vi "Xml_Load_Expert.vi"(7 "Version String":string, 8 "error in (no error)":errorcluster, 10 "XML Path":path=path "D:/TEST.xml", 11 "Refnum Clust":refnum<vi>) -> (0 "error out":errorcluster)   [LabVIEW 2024]
uses:
  controls/SOFTWARE_Inputs.ctl
  controls/HARDWARE_Inputs.ctl
  controls/AO_6711_Inputs.ctl
  controls/AO_6738_Inputs.ctl
  controls/AWG_5421_Inputs.ctl
  <instrlib>/niFgen/niFgen.llb/niFgen_ctl Trigger Source Values (Ring).ctl
  controls/DIGIT_5122_Inputs.ctl
  <instrlib>/niScope/Controls/niScope trigger source.ctl
  controls/HSDIO_6541_Inputs.ctl
  <instrlib>/niHSDIO/niHSDIO.llb/niHSDIO_ctl Trigger Source Values (Ring).ctl
  controls/EXPERT_Inputs.ctl
  controls/XML_Inputs.ctl
panel:
  in  "EXPERT Inputs":T1={"XML Inputs"={"Version Tag Name"="XML_Version", "Version String"="1.0"}, "SOFTWARE Inputs"={"Application Directory"=path "D:/S.O.F.T.S/LABVIEW/PIL", "Software Version"="1.0.0", "Data Path"=path "D:/PIRENEA/DATA", "XML Path"=path "D:/PIRENEA/DATA", "XML File Filter"="*.xml", "XML Saved Path"=path "D:/PIRENEA/DATA/SAVED", "Excit Scripts Path"=path "D:/PIRENEA/EXCIT_SCRIPTS", "Excit Scripts File Filter"="*.txt", "Excit Waveforms Path"=path "D:/PIRENEA/EXCIT_WFMS", "Excit Waveforms File Filter"="*.bin", "Timing Scripts Path"=path "D:/PIRENEA/TIMING_SCRIPTS", "Timing Scripts File Filter"="*.txt", "Timing Waveforms Path"=path "D:/PIRENEA/TIMING_WFMS", "Timing Waveforms File Filter"="*.bin", "Trapping Waveforms Path"=path "D:/PIRENEA/TRAPPING_WFMS", "Trapping Waveforms File Filter"="*.bin"}, "HSDIO 6541 Inputs"={"Resource Name"="HSDIO_6541", "Clock Rate"=1000000.0, "Trigger Source"="PFI0"}, "AWG 5421 Inputs"={"Resource Name"="AWG_5421", "Sample Rate"=10000000.0, "Trigger Type"=2, "Trigger Source"="PFI0", "Waveform Gain"=0.31, "Digital Filter ON"=TRUE}, "DIGIT 5122 Inputs"={"Sample Rate"=10000.0, "Resource Name"="DIGIT_5122", "Channel Name"="0", "Trigger Source"="VAL_EXTERNAL", "Vertical Range"=10.0, "Trigger Level"=3.0}, "AO 6711 Inputs"={"Physical Channels"="AO_6711/ao0:3", "Min Voltage"=-10.0, "Max Voltage"=10.0, "Trigger Source"="/AO_6711/PFI3", "Counter"="AO_6711/ctr0"}, "AO 6738 Inputs"={"Physical Channels"="AO_6738/ao0:3", "Min Voltage"=-10.0, "Max Voltage"=10.0, "Trigger Source"="/AO_6738/PFI2", "Counter"="AO_6738/ctr0"}} {"AO 6738 Inputs"."Max Voltage" min=-10.0 max=10.0; "AO 6738 Inputs"."Min Voltage" min=-10.0 max=10.0; "AWG 5421 Inputs"."Sample Rate" format="%.2p"; "AWG 5421 Inputs"."Trigger Type" items=["None", "Software Edge", "Digital Edge", "Digital Level"]; "AO 6711 Inputs"."Max Voltage" min=-10.0 max=10.0; "AO 6711 Inputs"."Min Voltage" min=-10.0 max=10.0; "HSDIO 6541 Inputs"."Clock Rate" format="%.2p"; "DIGIT 5122 Inputs"."Trigger Level" format="%.2f"; "DIGIT 5122 Inputs"."Vertical Range" format="%.2f"; "DIGIT 5122 Inputs"."Sample Rate" step=65535.0 format="%#_3p"}
  in  "HARDWARE Inputs":T12={"AO 6711 Inputs"={"Physical Channels"="AO_6711/ao0:3", "Min Voltage"=-10.0, "Max Voltage"=10.0, "Trigger Source"="/AO_6711/PFI3", "Counter"="AO_6711/ctr0"}, "AO 6738 Inputs"={"Physical Channels"="AO_6738/ao0:3", "Min Voltage"=-10.0, "Max Voltage"=10.0, "Trigger Source"="/AO_6738/PFI2", "Counter"="AO_6738/ctr0"}, "AWG 5421 Inputs"={"Resource Name"="AWG_5421", "Sample Rate"=10000000.0, "Trigger Type"=2, "Trigger Source"="PFI0", "Waveform Gain"=0.31, "Digital Filter ON"=TRUE}, "DIGIT 5122 Inputs"={"Sample Rate"=10000.0, "Resource Name"="DIGIT_5122", "Channel Name"="0", "Trigger Source"="VAL_EXTERNAL", "Vertical Range"=10.0, "Trigger Level"=3.0}, "HSDIO 6541 Inputs"={"Resource Name"="HSDIO_6541", "Clock Rate"=1000000.0, "Trigger Source"="PFI0"}} {"AO 6738 Inputs"."Max Voltage" min=-10.0 max=10.0; "AO 6738 Inputs"."Min Voltage" min=-10.0 max=10.0; "HSDIO 6541 Inputs"."Clock Rate" format="%.2p"; "DIGIT 5122 Inputs"."Trigger Level" format="%.2f"; "DIGIT 5122 Inputs"."Vertical Range" format="%.2f"; "DIGIT 5122 Inputs"."Sample Rate" step=65535.0 format="%#_3p"; "AWG 5421 Inputs"."Sample Rate" format="%.2p"; "AWG 5421 Inputs"."Trigger Type" items=["None", "Software Edge", "Digital Edge", "Digital Level"]; "AO 6711 Inputs"."Max Voltage" min=-10.0 max=10.0; "AO 6711 Inputs"."Min Voltage" min=-10.0 max=10.0}
  in  "SOFTWARE Inputs":T3={"Application Directory"=path "D:/S.O.F.T.S/LABVIEW/PIL", "Software Version"="1.0.0", "Data Path"=path "D:/PIRENEA/DATA", "XML Path"=path "D:/PIRENEA/DATA", "XML File Filter"="*.xml", "XML Saved Path"=path "D:/PIRENEA/DATA/SAVED", "Excit Scripts Path"=path "D:/PIRENEA/EXCIT_SCRIPTS", "Excit Scripts File Filter"="*.txt", "Excit Waveforms Path"=path "D:/PIRENEA/EXCIT_WFMS", "Excit Waveforms File Filter"="*.bin", "Timing Scripts Path"=path "D:/PIRENEA/TIMING_SCRIPTS", "Timing Scripts File Filter"="*.txt", "Timing Waveforms Path"=path "D:/PIRENEA/TIMING_WFMS", "Timing Waveforms File Filter"="*.bin", "Trapping Waveforms Path"=path "D:/PIRENEA/TRAPPING_WFMS", "Trapping Waveforms File Filter"="*.bin"}
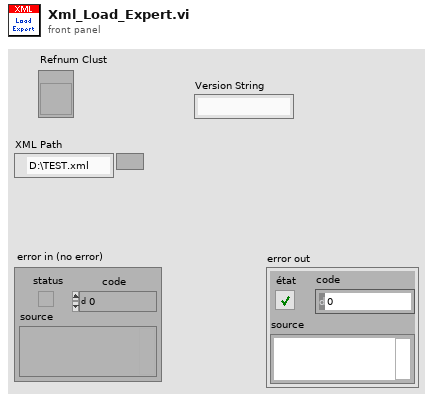
[diagram p1: front panel]
types:
  T1 = typedef "EXPERT_Inputs.ctl" = cluster{"XML Inputs":T2, "SOFTWARE Inputs":T3, "HSDIO 6541 Inputs":T4, "AWG 5421 Inputs":T6, "DIGIT 5122 Inputs":T8, "AO 6711 Inputs":T10, "AO 6738 Inputs":T11}
  T2 = typedef "XML_Inputs.ctl" = cluster{"Version Tag Name":string, "Version String":string}
  T3 = typedef "SOFTWARE_Inputs.ctl" = cluster{"Application Directory":path, "Software Version":string, "Data Path":path, "XML Path":path, "XML File Filter":string, "XML Saved Path":path, "Excit Scripts Path":path, "Excit Scripts File Filter":string, "Excit Waveforms Path":path, "Excit Waveforms File Filter":string, "Timing Scripts Path":path, "Timing Scripts File Filter":string, "Timing Waveforms Path":path, "Timing Waveforms File Filter":string, "Trapping Waveforms Path":path, "Trapping Waveforms File Filter":string}
  T4 = typedef "HSDIO_6541_Inputs.ctl" = cluster{"Resource Name":refnum<k15>, "Clock Rate":dbl, "Trigger Source":T5}
  T5 = typedef "niHSDIO_ctl Trigger Source Values (Ring).ctl" = string
  T6 = typedef "AWG_5421_Inputs.ctl" = cluster{"Resource Name":refnum<k15>, "Sample Rate":dbl, "Trigger Type":u16, "Trigger Source":T7, "Waveform Gain":dbl, "Digital Filter ON":bool}
  T7 = typedef "niFgen_ctl Trigger Source Values (Ring).ctl" = string
  T8 = typedef "DIGIT_5122_Inputs.ctl" = cluster{"Sample Rate":dbl, "Resource Name":refnum<k15>, "Channel Name":string, "Trigger Source":T9, "Vertical Range":dbl, "Trigger Level":dbl}
  T9 = typedef "niScope trigger source.ctl" = string
  T10 = typedef "AO_6711_Inputs.ctl" = cluster{"Physical Channels":tag, "Min Voltage":dbl, "Max Voltage":dbl, "Trigger Source":tag, "Counter":tag}
  T11 = typedef "AO_6738_Inputs.ctl" = cluster{"Physical Channels":tag, "Min Voltage":dbl, "Max Voltage":dbl, "Trigger Source":tag, "Counter":tag}
  T12 = typedef "HARDWARE_Inputs.ctl" = cluster{"AO 6711 Inputs":T10, "AO 6738 Inputs":T11, "AWG 5421 Inputs":T6, "DIGIT 5122 Inputs":T8, "HSDIO 6541 Inputs":T4}
  T13 = cluster{"Application Directory":path, "Resources Path":path, "Data Path":path, "XML Path":path, "XML File Filter":string, "Excit Scripts Path":path, "Excit Scripts File Filter":string, "Excit Waveforms Path":path, "Excit Waveforms File Filter":string, "Timing Scripts Path":path, "Timing Scripts File Filter":string, "Timing Waveforms Path":path, "Timing Waveforms File Filter":string, "Trapping Waveforms Path":path, "Trapping Waveforms File Filter":string}
  T14 = cluster{"Physical Channels":tag, "Min Voltage":dbl, "Max Voltage":dbl, "Trigger Source":tag, "Counter":tag}
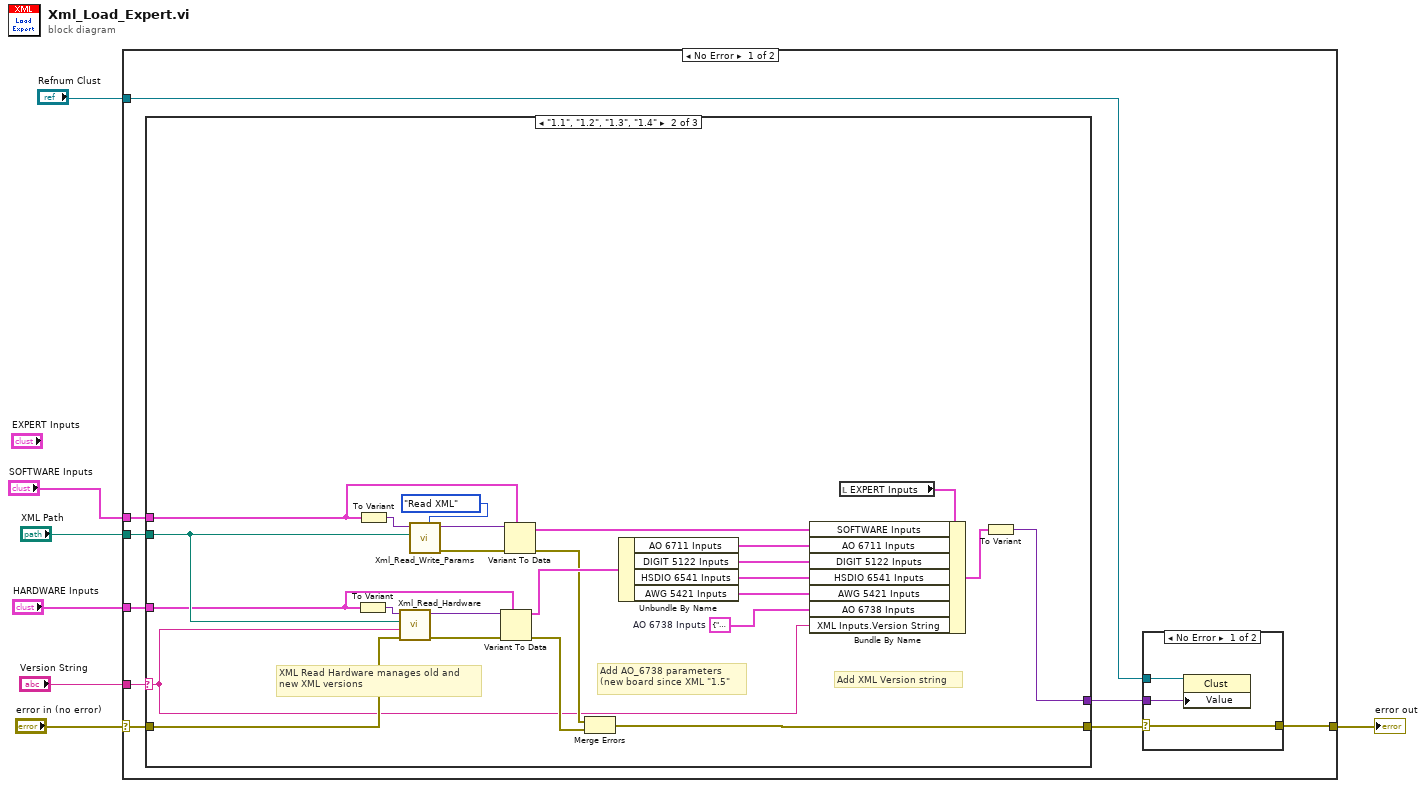
[diagram p0: block diagram]
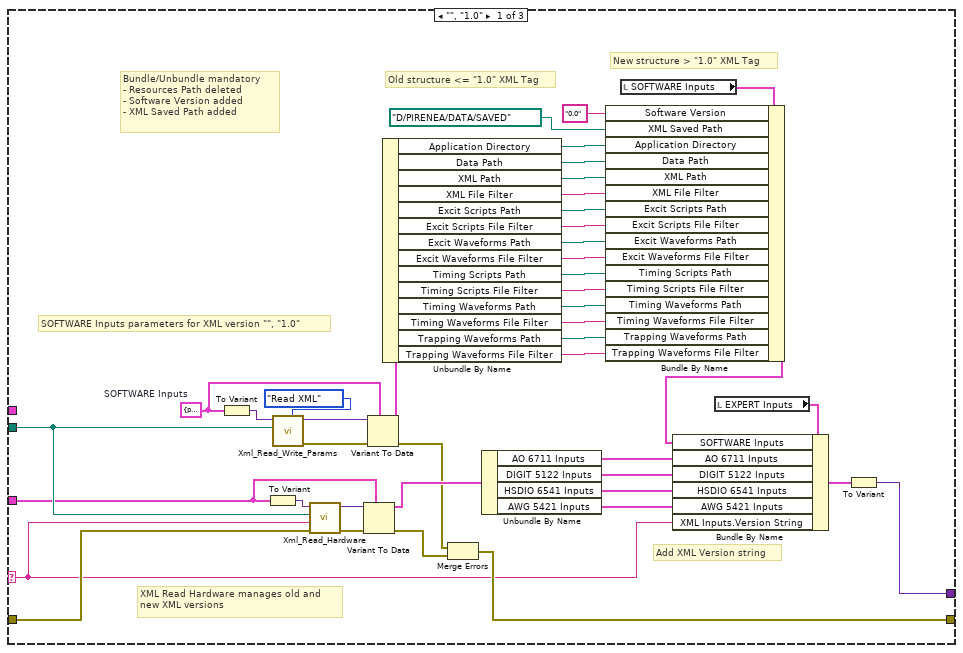
[diagram p3: hidden frame]
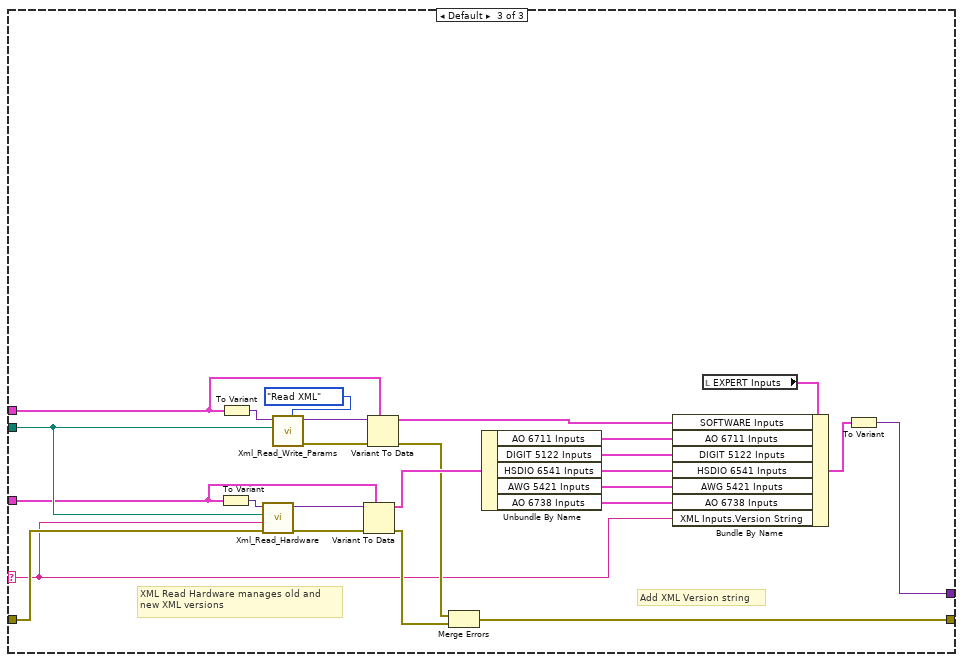
[diagram p4: hidden frame]
diagram:
  n1 = case shown="No Error" "error in (no error)" {
    selector: "error in (no error)" -> [w16 w113]
    tunnel: "XML Path" -> [w15 _]
    tunnel: [w12 w113] -> w5
    tunnel: "Version String" -> [w14 _]
    tunnel: "Refnum Clust" -> [w10 _]
    tunnel: "HARDWARE Inputs" -> [w9 _]
    tunnel: "SOFTWARE Inputs" -> [w8 _]
    frame No Error {
      n2 = case shown="\"1.1\", \"1.2\", \"1.3\", \"1.4\"" w14 {
        selector: w14 -> [w43 w64 w92]
        tunnel: w16 -> [w44 w68 w93]
        tunnel: w15 -> [w62 w87 w112]
        tunnel: [w50 w74 w99] -> w11
        tunnel: [w47 w71 w96] -> w13
        tunnel: w9 -> [w21 w66 w90]
        tunnel: w8 -> [_ w65 w89]
        frame "", "1.0" {
          w42 = T13 {"Application Directory"=path "D:/S.O.F.T.S/LABVIEW/PIL", "Resources Path"=path "", "Data Path"=path "D:/PIRENEA/DATA", "XML Path"=path "D:/PIRENEA/DATA", "XML File Filter"="*.xml", "Excit Scripts Path"=path "D:/PIRENEA/EXCIT_SCRIPTS", "Excit Scripts File Filter"="*.txt", "Excit Waveforms Path"=path "D:/PIRENEA/EXCIT_WFMS", "Excit Waveforms File Filter"="*.bin", "Timing Scripts Path"=path "D:/PIRENEA/TIMING_SCRIPTS", "Timing Scripts File Filter"="*.txt", "Timing Waveforms Path"=path "D:/PIRENEA/TIMING_WFMS", "Timing Waveforms File Filter"="*.bin", "Trapping Waveforms Path"=path "D:/PIRENEA/TRAPPING_WFMS", "Trapping Waveforms File Filter"="*.bin"}  # SOFTWARE Inputs
          # "New structure > \"1.0\" XML Tag"
          # "Old structure <= \"1.0\" XML Tag"
          # "Bundle/Unbundle mandatory\n- Resources Path deleted\n- Software Version added\n- XML Saved Path added"
          # "SOFTWARE Inputs parameters for XML version \"\", \"1.0\""
          # "XML Read Hardware manages old and\nnew XML versions"
          # "Add XML Version string"
          n3 = To Variant(anything=w42) -> (Variant=w61:variant)
          n4 = To Variant(anything=w21) -> (Variant=w45:variant)
          n5 = call "Xml_Read_Write_Params.vi"("Variant"=w61, "XML Path"=w62, "Command"=enum16{"Read XML", "Set", "Get", "Write XML"}."Read XML") -> ("Variant Output"=w59:variant, "error out"=w60:errorcluster)  [unwired: 4 in, 1 out]
          n6 = call "Xml_Read_Hardware.vi"("error in (no error)"=w44, "Version String"=w43, "XML Path"=w62, "Variant"=w45) -> ("error out"=w54:errorcluster, "Variant Output"=w53:variant)  [unwired: 6 in]
          n7 = Variant To Data(error in=w54, type=w21, Variant=w53) -> (data=w52:T12, error out=w49:errorcluster)
          n8 = Variant To Data(error in=w60, type=w42, Variant=w59) -> (data=w41:T13, error out=w48:errorcluster)
          n9 = Unbundle By Name(w41) -> ("Application Directory"=w24:path, "Data Path"=w28:path, "XML Path"=w29:path, "XML File Filter"=w30:string, "Excit Scripts Path"=w31:path, "Excit Scripts File Filter"=w32:string, "Excit Waveforms Path"=w33:path, "Excit Waveforms File Filter"=w34:string, "Timing Scripts Path"=w35:path, "Timing Scripts File Filter"=w36:string, "Timing Waveforms Path"=w37:path, "Timing Waveforms File Filter"=w38:string, "Trapping Waveforms Path"=w27:path, "Trapping Waveforms File Filter"=w26:string)
          n10 = Merge Errors(w48, w49) -> (w47:errorcluster)
          n11 = Unbundle By Name(w52) -> ("AO 6711 Inputs"=w57:T10, "DIGIT 5122 Inputs"=w56:T8, "HSDIO 6541 Inputs"=w55:T4, "AWG 5421 Inputs"=w46:T6)
          n12 = local read "SOFTWARE Inputs"() -> (w39:T3)
          n13 = Bundle By Name(cluster=w39, "Software Version"="0.0", "XML Saved Path"=path "D:/PIRENEA/DATA/SAVED", "Application Directory"=w24, "Data Path"=w28, "XML Path"=w29, "XML File Filter"=w30, "Excit Scripts Path"=w31, "Excit Scripts File Filter"=w32, "Excit Waveforms Path"=w33, "Excit Waveforms File Filter"=w34, "Timing Scripts Path"=w35, "Timing Scripts File Filter"=w36, "Timing Waveforms Path"=w37, "Timing Waveforms File Filter"=w38, "Trapping Waveforms Path"=w27, "Trapping Waveforms File Filter"=w26) -> (w25:T3)
          n14 = local read "EXPERT Inputs"() -> (w40:T1)
          n15 = Bundle By Name(cluster=w40, "SOFTWARE Inputs"=w25, "AO 6711 Inputs"=w57, "DIGIT 5122 Inputs"=w56, "HSDIO 6541 Inputs"=w55, "AWG 5421 Inputs"=w46, "XML Inputs.Version String"=w43) -> (w51:T1)
          n16 = To Variant(anything=w51) -> (Variant=w50:variant)
        }
        frame "1.1", "1.2", "1.3", "1.4" {
          w63 = T14 {"Physical Channels"="AO_6738/ao0:3", "Min Voltage"=-10.0, "Max Voltage"=10.0, "Trigger Source"="/AO_6738/PFI2", "Counter"="AO_6738/ctr0"}  # AO 6738 Inputs
          # "Add AO_6738 parameters\n(new board since XML \"1.5\""
          # "XML Read Hardware manages old and\nnew XML versions"
          # "Add XML Version string"
          n17 = To Variant(anything=w66) -> (Variant=w69:variant)
          n18 = To Variant(anything=w65) -> (Variant=w86:variant)
          n19 = call "Xml_Read_Hardware.vi"("error in (no error)"=w68, "Version String"=w64, "XML Path"=w87, "Variant"=w69) -> ("error out"=w78:errorcluster, "Variant Output"=w77:variant)  [unwired: 6 in]
          n20 = call "Xml_Read_Write_Params.vi"("Variant"=w86, "XML Path"=w87, "Command"=enum16{"Read XML", "Set", "Get", "Write XML"}."Read XML") -> ("Variant Output"=w84:variant, "error out"=w85:errorcluster)  [unwired: 4 in, 1 out]
          n21 = Variant To Data(error in=w78, type=w66, Variant=w77) -> (data=w76:T12, error out=w73:errorcluster)
          n22 = Variant To Data(error in=w85, type=w65, Variant=w84) -> (data=w82:T3, error out=w72:errorcluster)
          n23 = Merge Errors(w72, w73) -> (w71:errorcluster)
          n24 = Unbundle By Name(w76) -> ("AO 6711 Inputs"=w81:T10, "DIGIT 5122 Inputs"=w80:T8, "HSDIO 6541 Inputs"=w79:T4, "AWG 5421 Inputs"=w70:T6)
          n25 = local read "EXPERT Inputs"() -> (w67:T1)
          n26 = Bundle By Name(cluster=w67, "SOFTWARE Inputs"=w82, "AO 6711 Inputs"=w81, "DIGIT 5122 Inputs"=w80, "HSDIO 6541 Inputs"=w79, "AWG 5421 Inputs"=w70, "AO 6738 Inputs"=w63, "XML Inputs.Version String"=w64) -> (w75:T1)
          n27 = To Variant(anything=w75) -> (Variant=w74:variant)
        }
        frame Default {
          # "XML Read Hardware manages old and\nnew XML versions"
          # "Add XML Version string"
          n28 = To Variant(anything=w90) -> (Variant=w94:variant)
          n29 = To Variant(anything=w89) -> (Variant=w111:variant)
          n30 = call "Xml_Read_Hardware.vi"("error in (no error)"=w93, "Version String"=w92, "XML Path"=w112, "Variant"=w94) -> ("error out"=w103:errorcluster, "Variant Output"=w102:variant)  [unwired: 6 in]
          n31 = call "Xml_Read_Write_Params.vi"("Variant"=w111, "XML Path"=w112, "Command"=enum16{"Read XML", "Set", "Get", "Write XML"}."Read XML") -> ("Variant Output"=w109:variant, "error out"=w110:errorcluster)  [unwired: 4 in, 1 out]
          n32 = Variant To Data(error in=w103, type=w90, Variant=w102) -> (data=w101:T12, error out=w98:errorcluster)
          n33 = Variant To Data(error in=w110, type=w89, Variant=w109) -> (data=w107:T3, error out=w97:errorcluster)
          n34 = Merge Errors(w97, w98) -> (w96:errorcluster)
          n35 = Unbundle By Name(w101) -> ("AO 6711 Inputs"=w106:T10, "DIGIT 5122 Inputs"=w105:T8, "HSDIO 6541 Inputs"=w104:T4, "AWG 5421 Inputs"=w95:T6, "AO 6738 Inputs"=w88:T11)
          n36 = local read "EXPERT Inputs"() -> (w91:T1)
          n37 = Bundle By Name(cluster=w91, "SOFTWARE Inputs"=w107, "AO 6711 Inputs"=w106, "DIGIT 5122 Inputs"=w105, "HSDIO 6541 Inputs"=w104, "AWG 5421 Inputs"=w95, "AO 6738 Inputs"=w88, "XML Inputs.Version String"=w92) -> (w100:T1)
          n38 = To Variant(anything=w100) -> (Variant=w99:variant)
        }
      }
      n39 = case shown="No Error" w13 {
        selector: w13 -> [w18 w20]
        tunnel: w10 -> [w19 _]
        tunnel: [w18 w20] -> w12
        tunnel: w11 -> [w17 _]
        frame No Error {
          n40 = property class="Clust"(reference=w19, "Value"=w17) -> ()  [unwired: 1 in, 2 out]
        }
        frame Error {
        }
      }
    }
    frame Error {
    }
  }
  "error out" <- w5
